vi "Condition jsObject Array.vi"(7 "Connection Refnum":T1, 8 "error in (no error)":errorcluster, 9 "CONDITIONS (none)":T2[](array[typedef])) -> (0 "error out":errorcluster, 2 "Conditions jsObject Array":string, 5 "dup Connection Refnum":T1)   [LabVIEW 2011]
uses:
  Condition Record.ctl
  Condition Operators.ctl
  SI.LIB/ODBC/SQL Controls/Connection Refnum.ctl
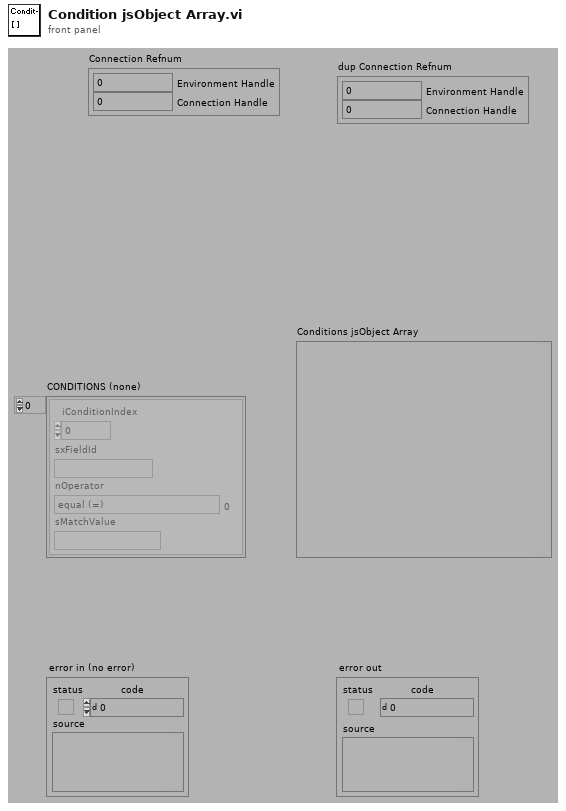
[diagram p1: front panel]
types:
  T1 = typedef "Connection Refnum.ctl" = cluster{"Environment Handle":i32, "Connection Handle":i32}
  T2 = typedef "Condition Record.ctl" = cluster{"iConditionIndex":i32, "sxFieldId":string, "nOperator":T3, "sMatchValue":string}
  T3 = typedef "Condition Operators.ctl" = enum16{"equal (=)", "not equal (\\u2260)", "less than (<)", "less than or equal (\\u2264)", "greater than (>)", "greater than or equal (\\u2265)", "contains", "does not contain"}
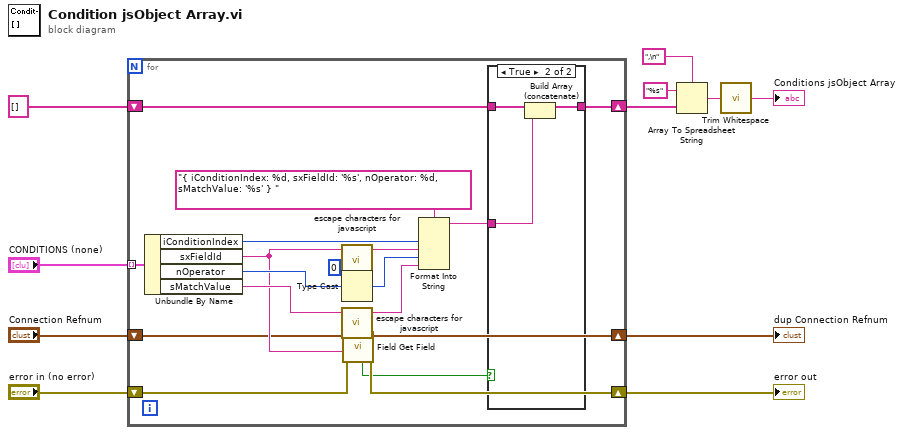
[diagram p0: block diagram]
diagram:
  n1 = for {
    shift-right: [w17] -> w9
    shift-left: "error in (no error)" -> [w23]
    tunnel: "CONDITIONS (none)" -> [w24] mode=indexing
    shift-right: [w16] -> w6
    shift-left: "Connection Refnum" -> [w18]
    shift-right: [w13] -> w1
    shift-left: string[] [] -> [w14]
    n2 = Unbundle By Name(w24) -> ("iConditionIndex"=w22:i32, "sxFieldId"=w19:string, "nOperator"=w27:T3, "sMatchValue"=w28:string)
    n3 = call "escape characters for javascript.vi"("String (\"\")"=w19) -> ("escaped String"=w21:string)  [unwired: 4 out]
    n4 = Type Cast(type=u16 0, x=w27) -> (*(type *) &x=w20:u16)
    n5 = call "escape characters for javascript.vi"("String (\"\")"=w28) -> ("escaped String"=w29:string)  [unwired: 4 out]
    n6 = call "Field Get Field.vi"("error in (no error)"=w23, "sFieldId or sDisplayName (\"\")"=w19, "Connection Refnum"=w18) -> ("error out"=w17:errorcluster, "Connection Refnum"=w16:T1, "Data Present?"=w15:bool)  [unwired: 2 in, 4 out]
    n7 = Format Into String(format string="{ iConditionIndex: %d, sxFieldId: '%s', nOperator: %d, sMatchValue: '%s' } ", w22, w21, w20, w29) -> (resulting string=w12:string)  [unwired: 2 in, 1 out]
    n8 = case shown="True" w15 {
      tunnel: w14 -> [w30 w33]
      tunnel: [w30 w32] -> w13
      tunnel: w12 -> [_ w31]
      frame False {
      }
      frame True {
        n9 = Build Array (concatenate)(w33, w31) -> (w32:string[])
      }
    }
  }
  "error out" <- w9
  "dup Connection Refnum" <- w6
  n10 = Array To Spreadsheet String(delimiter (Tab)=",\n", array=w1, 3:"%s" ("format string")) -> (spreadsheet string=w3:string)
  n11 = call <vilib>:"Trim Whitespace.vi"("string"=w3) -> ("trimmed string"=→"Conditions jsObject Array":string)  [unwired: 1 in]
